vi "Section selection.vi"(4 "Length":i32, 7 "Event final":dbl[][](array[numeric])) -> (3 "Distribution (output)":T1)   [LabVIEW 2017]
uses:
  <vilib>/Analysis/NI_AALBase.lvlib
  <vilib>/Analysis/NI_AALPro.lvlib
panel:
  out "Mean Frequency":string
  out "EVT #":string caption="String"
  out "Mean Amplitude":string caption="String"
  out "Mean IEI":string caption="String"
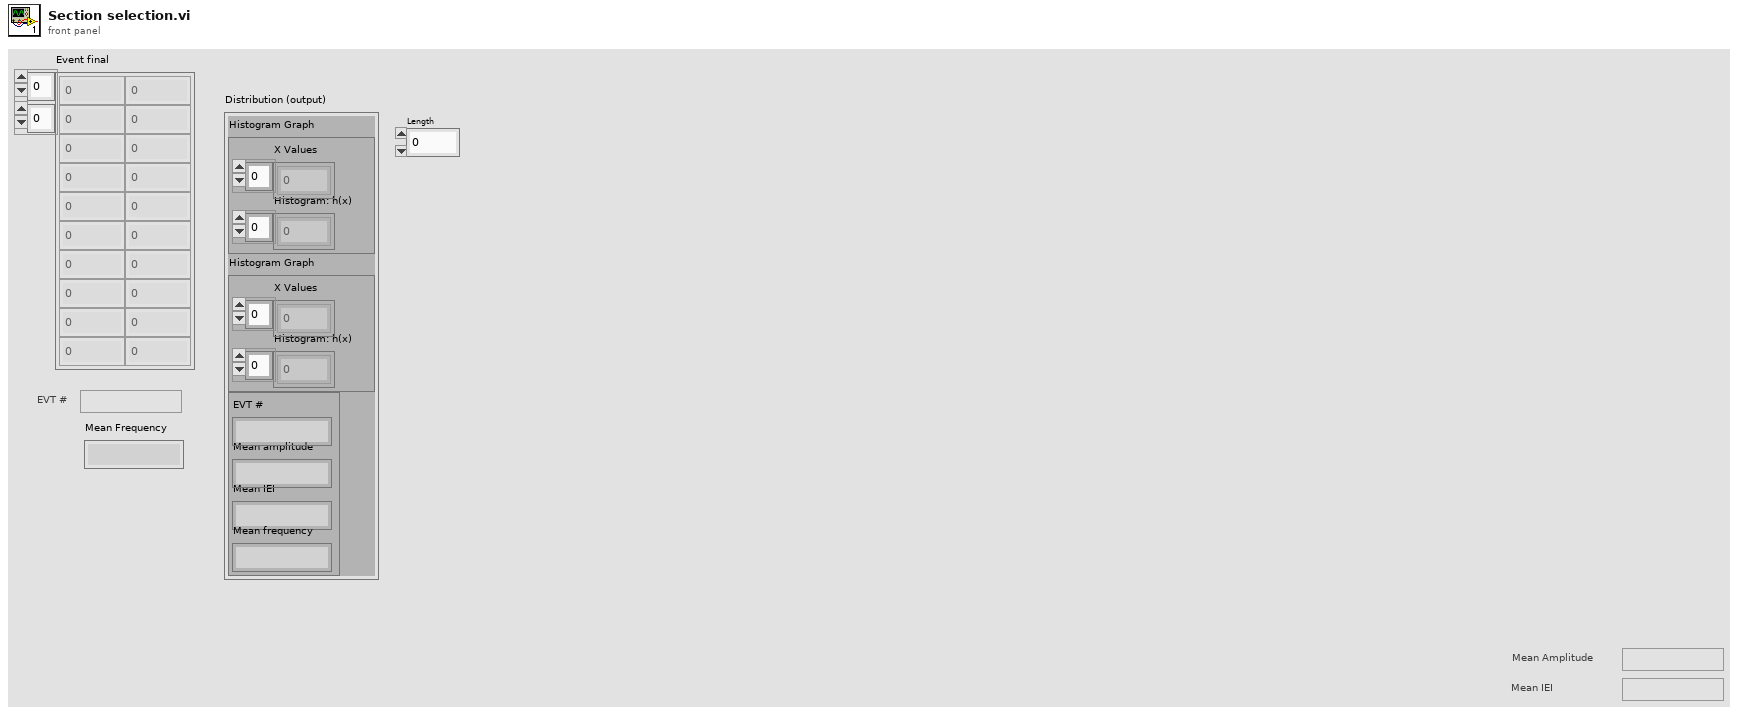
[diagram p1: front panel]
types:
  T1 = cluster{"Histogram Graph":cluster{"X Values":dbl[], "Histogram: h(x)":i32[]}, "Histogram Graph":cluster{"X Values":dbl[], "Histogram: h(x)":i32[]}, cluster{"EVT #":string, "Mean amplitude":string, "Mean IEI":string, "Mean frequency":string}}
  T2 = cluster{string, "standard deviation":string, "standard deviation":string, string}
  T3 = cluster{"X Values":dbl[], "Histogram: h(x)":i32[]}
  T4 = cluster{"Histogram Graph":cluster{"X Values":dbl[], "Histogram: h(x)":i32[]}, "Histogram Graph":cluster{"X Values":dbl[], "Histogram: h(x)":i32[]}, cluster{string, "standard deviation":string, "standard deviation":string, string}}
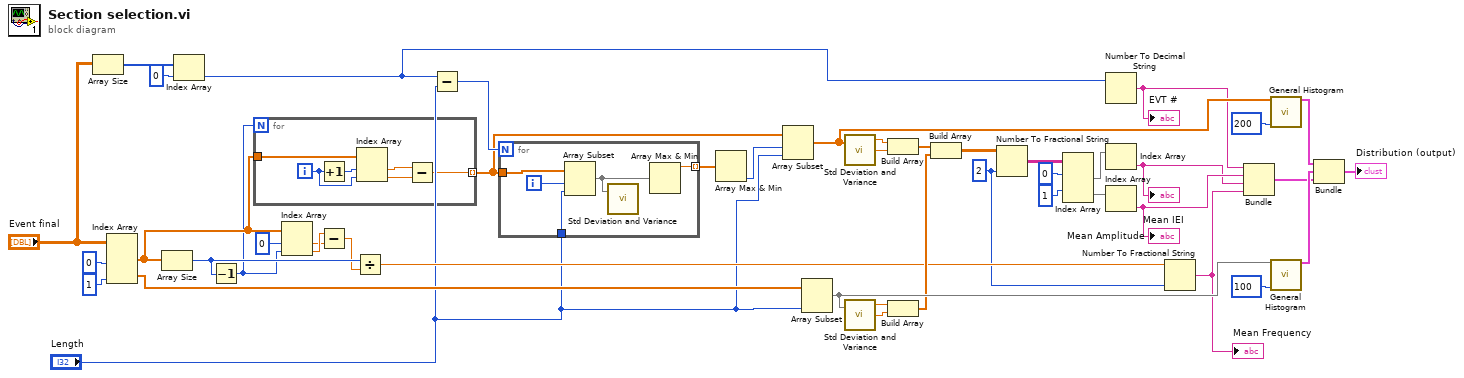
[diagram p0: block diagram]
diagram:
  w3 = i16 2 ("폭(-)")
  n1 = Array Size(array="Event final") -> (size(s)=w45:i32[])
  n2 = Index Array(array="Event final", index (col) #1=0 ("비활성화된 인덱스 (열)"), index (col) #2=1 ("인덱스 (열)")) -> (element #1=w13:dbl[], element #2=w37:dbl[])  [unwired: 2 in]
  n3 = Array Size(array=w13) -> (size(s)=w9:i32)
  n4 = Index Array(array=w45, index=0 ("인덱스")) -> (element=w1:i32)
  n5 = Decrement(x=w9) -> (x-1=w4:i32)
  n6 = for {
    N: w4 -> [_]
    tunnel: w13 -> [w51]
    tunnel: [w46] -> w38 mode=indexing
    i -> [w49]
    n7 = Increment(x=w49) -> (x+1=w50:i32)
    n8 = Index Array(array=w51, index #1=w50, index #2=w49) -> (element #1=w48:dbl, element #2=w47:dbl)
    n9 = Subtract(x=w48, y=w47) -> (x-y=w46:dbl)
  }
  n10 = Index Array(array=w13, index #1=0 ("인덱스"), index #2=w4) -> (element #1=w10:dbl, element #2=w11:dbl)
  n11 = Subtract(x=w11, y=w10) -> (x-y=w8:dbl)
  n12 = Divide(x=w9, y=w8) -> (x/y=w7:dbl)
  n13 = Subtract(x=w1, y="Length") -> (x-y=w43:i32)
  n14 = for {
    N: w43 -> [_]
    tunnel: w38 -> [w56]
    tunnel: [w53] -> w40 mode=indexing
    tunnel: "Length" -> [w52]
    i -> [w55]
    n15 = Array Subset(array=w56, index=w55, length=w52) -> (w54:dbl[])
    n16 = call <vilib>:"Std Deviation and Variance.vi"("X"=w54) -> ()  [unwired: 1 in, 3 out]
    n17 = Array Max & Min(array=w54) -> (max value=w53:dbl)  [unwired: 3 out]
  }
  n18 = Array Max & Min(array=w40) -> (min index (indices)=w26:i32)  [unwired: 3 out]
  n19 = Array Subset(array=w38, index=w26, length="Length") -> (w34:dbl[])
  n20 = Array Subset(array=w37, length="Length") -> (w33:dbl[])  [unwired: 1 in]
  n21 = call <vilib>:"Std Deviation and Variance.vi"("X"=w34) -> ("mean"=w32:dbl, "standard deviation"=w31:dbl)  [unwired: 1 in, 1 out]
  n22 = call <vilib>:"Std Deviation and Variance.vi"("X"=w33) -> ("mean"=w30:dbl, "standard deviation"=w29:dbl)  [unwired: 1 in, 1 out]
  n23 = Build Array(w32, w31) -> (w28:dbl[])
  n24 = Build Array(w30, w29) -> (w27:dbl[])
  n25 = Build Array(w28, w27) -> (w25:dbl[][])
  n26 = Number To Fractional String(number=w25, precision (6)=w3) -> (F-format string=w24:string[][])  [unwired: 2 in]
  n27 = Index Array(array=w24, index (row) #1=0 ("인덱스 (행)"), index (row) #2=1 ("인덱스 (행)")) -> (element #1=w21:string[], element #2=w20:string[])  [unwired: 2 in]
  n28 = Number To Decimal String(number=w1) -> (decimal integer string=w17:string)  [unwired: 1 in]
  "EVT #" <- w17
  n29 = Index Array(array=w21) -> (element=w14:string)  [unwired: 1 in]
  "Mean IEI" <- w14
  n30 = Index Array(array=w20) -> (element=w15:string)  [unwired: 1 in]
  "Mean Amplitude" <- w15
  n31 = Number To Fractional String(number=w7, precision (6)=w3) -> (F-format string=w6:string)  [unwired: 2 in]
  "Mean Frequency" <- w6
  n32 = Bundle(w17, "standard deviation"=w15, "standard deviation"=w14, w6) -> (w16:T2)  [unwired: 1 in]
  n33 = call <vilib>:"General Histogram.vi"("X"=w34, "# bins"=200) -> ("Histogram Graph"=w19:T3)  [unwired: 9 in, 4 out]
  n34 = call <vilib>:"General Histogram.vi"("X"=w33, "# bins"=100) -> ("Histogram Graph"=w18:T3)  [unwired: 9 in, 4 out]
  n35 = Bundle("Histogram Graph"=w19, "Histogram Graph"=w18, w16) -> (→"Distribution (output)":T4)  [unwired: 1 in]
